vi "orrd.vi"(8 "arreglo modificado":string[](array[string]), 9 "Arreglo dim":bool[](array[boolean]), 10 "entrada":string, 11 "arreglo entrada":string[](array[string])) -> (2 "salida":string)   [LabVIEW 2016]
panel:
  out "String":string
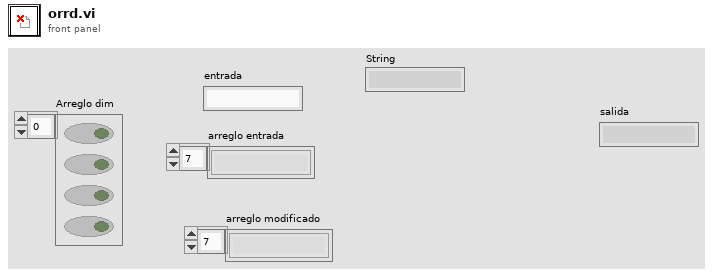
[diagram p1: front panel]
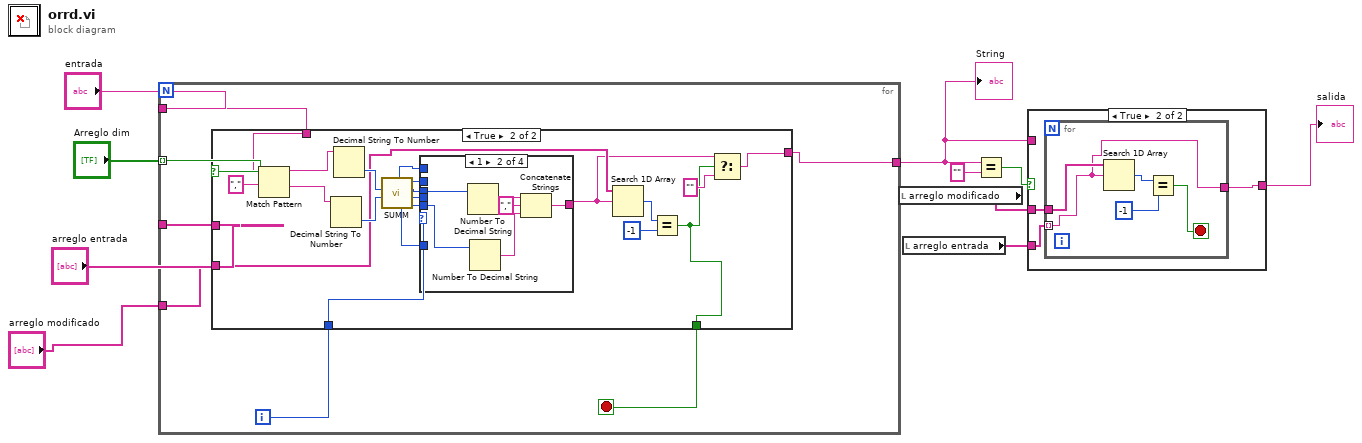
[diagram p0: block diagram]
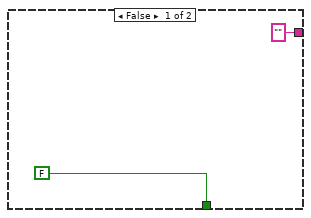
[diagram p3: hidden frame]
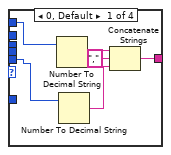
[diagram p4: hidden frame]
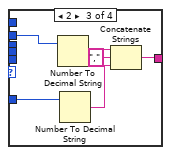
[diagram p5: hidden frame]
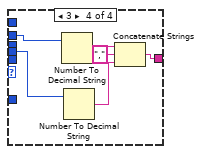
[diagram p6: hidden frame]
diagram:
  n1 = for {
    tunnel: "Arreglo dim" -> [w17] mode=indexing
    tunnel: "entrada" -> [w13]
    tunnel: "arreglo entrada" -> [w15]
    tunnel: "arreglo modificado" -> [w12]
    tunnel: [w11] -> w3
    i -> [w14]
    stop <- w16 stop-if-true
    n2 = case shown="True" w17 {
      tunnel: [FALSE w20] -> w16
      tunnel: w15 -> [_ _]
      tunnel: w14 -> [_ w39]
      tunnel: w13 -> [_ w38]
      tunnel: w12 -> [_ w26]
      tunnel: ["" w23] -> w11
      frame False {
      }
      frame True {
        n3 = Match Pattern(string=w38, regular expression=",") -> (before substring=w36:string, after substring=w35:string)  [unwired: 1 in, 2 out]
        n4 = Decimal String To Number(string=w35) -> (number=w33:i32)  [unwired: 2 in, 1 out]
        n5 = Decimal String To Number(string=w36) -> (number=w34:i32)  [unwired: 2 in, 1 out]
        n6 = call "SUMM.vi"("Y"=w33, "X"=w34) -> ("Y"=w32:i32, "Y+1"=w27:i32, "X+1"=w30:i32, "X"=w29:i32, "Y-1"=w28:i32, "X-1"=w31:i32)  [unwired: 4 in]
        n7 = case shown="1" w39 {
          tunnel: w32 -> [w44 w48 _ _]
          tunnel: w31 -> [w45 _ _ _]
          tunnel: [w41 w46 w54 w60] -> w21
          tunnel: w30 -> [_ w47 _ _]
          tunnel: w29 -> [_ _ w53 w59]
          tunnel: w28 -> [_ _ w52 _]
          tunnel: w27 -> [_ _ _ w58]
          frame 0, Default {
            n8 = Number To Decimal String(number=w45) -> (decimal integer string=w43:string)  [unwired: 1 in]
            n9 = Number To Decimal String(number=w44) -> (decimal integer string=w42:string)  [unwired: 1 in]
            n10 = Concatenate Strings(w43, "," ("string"), w42) -> (w41:string)
          }
          frame 1 {
            n11 = Number To Decimal String(number=w47) -> (decimal integer string=w51:string)  [unwired: 1 in]
            n12 = Number To Decimal String(number=w48) -> (decimal integer string=w50:string)  [unwired: 1 in]
            n13 = Concatenate Strings(w51, "," ("string"), w50) -> (w46:string)
          }
          frame 2 {
            n14 = Number To Decimal String(number=w53) -> (decimal integer string=w57:string)  [unwired: 1 in]
            n15 = Number To Decimal String(number=w52) -> (decimal integer string=w56:string)  [unwired: 1 in]
            n16 = Concatenate Strings(w57, "," ("string"), w56) -> (w54:string)
          }
          frame 3 {
            n17 = Number To Decimal String(number=w59) -> (decimal integer string=w63:string)  [unwired: 1 in]
            n18 = Number To Decimal String(number=w58) -> (decimal integer string=w62:string)  [unwired: 1 in]
            n19 = Concatenate Strings(w63, "," ("string"), w62) -> (w60:string)
          }
        }
        n20 = Search 1D Array(1D array=w26, element=w21) -> (index of element=w25:i32)  [unwired: 1 in]
        n21 = Equal?(x=w25, y=-1) -> (x = y?=w20:bool)
        n22 = Select(t=w21, s=w20, f="") -> (s? t:f=w23:string)
      }
    }
  }
  "String" <- w3
  n23 = local read "arreglo modificado"() -> (w2:string[])
  n24 = local read "arreglo entrada"() -> (w1:string[])
  n25 = Equal?(x=w3, y="") -> (x = y?=w5:bool)
  n26 = case shown="True" w5 {
    tunnel: [w64 w65] -> w4
    tunnel: w3 -> [w64 _]
    tunnel: w2 -> [_ w67]
    tunnel: w1 -> [_ w66]
    frame False {
    }
    frame True {
      n27 = for {
        tunnel: w67 -> [w72]
        tunnel: w66 -> [w68] mode=indexing
        tunnel: [w68] -> w65
        stop <- w69 stop-if-true
        n28 = Search 1D Array(1D array=w72, element=w68) -> (index of element=w71:i32)  [unwired: 1 in]
        n29 = Equal?(x=w71, y=-1) -> (x = y?=w69:bool)
      }
    }
  }
  "salida" <- w4
